vi "Cp.vi"(9 "l":dbl, 10 "beta":dbl, 11 "alpha":dbl) -> (3 "Array":dbl[](array[numeric]))   [LabVIEW 2011]
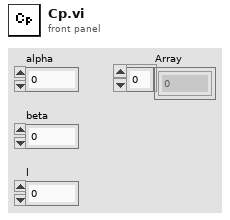
[diagram p1: front panel]
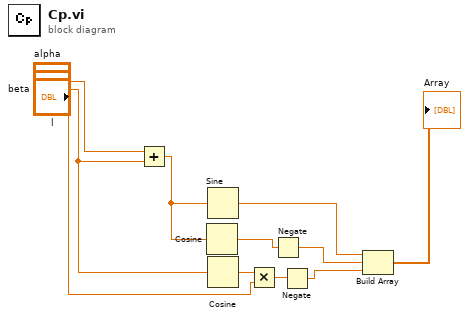
[diagram p0: block diagram]
diagram:
  n1 = Add(x="alpha", y="beta") -> (x+y=w2:dbl)
  n2 = Cosine(x=w2) -> (cos(x)=w7:dbl)
  n3 = Sine(x=w2) -> (sin(x)=w10:dbl)
  n4 = Cosine(x="beta") -> (cos(x)=w4:dbl)
  n5 = Multiply(x=w4, y="l") -> (x*y=w6:dbl)
  n6 = Negate(x=w7) -> (-x=w9:dbl)
  n7 = Negate(x=w6) -> (-x=w8:dbl)
  n8 = Build Array(w10, w9, w8) -> (→"Array":dbl[])
